vi "append_to_log.vi"(5 "data_type":T1, 7 "dims":T2, 8 "error in (no error)":errorcluster, 9 "Location":string, 10 "Data":variant, 11 "scan_hdf5_log in":refnum<class "scan_hdf5_log.lvclass">) -> (0 "error out":errorcluster, 3 "scan_hdf5_log out":refnum<class "scan_hdf5_log.lvclass">)   [LabVIEW 2015, in "scan_hdf5_log.lvclass"]
uses:
  scan_hdf5_log.lvclass
  Data Logger Class/data_dimensionality.ctl
  Data Logger Class/logger_data_types.ctl
  scan_hdf5_log.lvclass/scan_hdf5_log.ctl
  <vilib>/UPVI/lvhdf5/dataset.llb/Append Element(s) to Dataset (Variant).vi
  <vilib>/UPVI/lvhdf5/dataset.llb/Append Element(s) to Dataset.xnode
  <vilib>/UPVI/lvhdf5/library.llb/HDF5 Ref.ctl
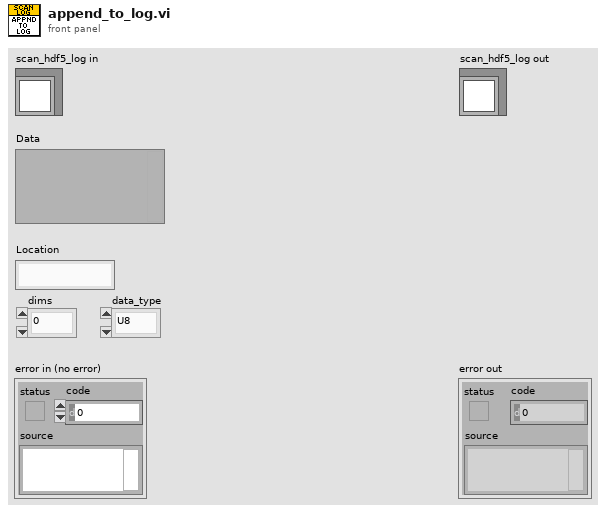
[diagram p1: front panel]
types:
  T1 = typedef "logger_data_types.ctl" = enum16{"U8", "I8", "U16", "I16", "U32", "I32", "DBL", "String"}
  T2 = typedef "data_dimensionality.ctl" = enum16{"0", "1", "2"}
  T3 = typedef "HDF5 Ref.ctl" = refnum<k1>
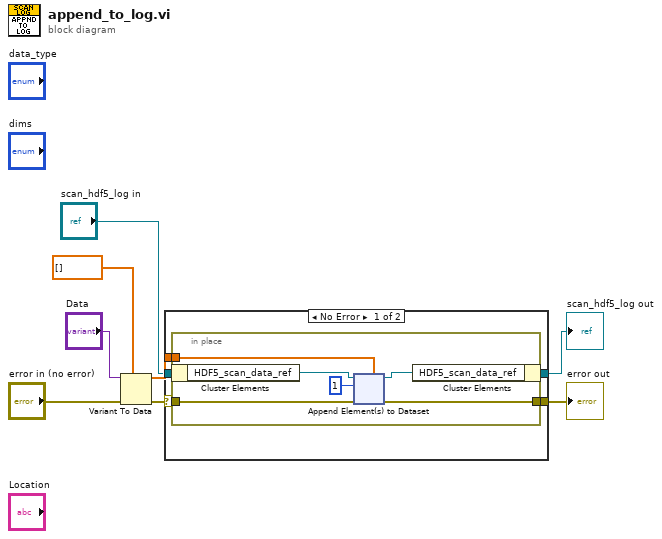
[diagram p0: block diagram]
diagram:
  n1 = Variant To Data(error in="error in (no error)", type=dbl[] [], Variant="Data") -> (data=w5:dbl[], error out=w4:errorcluster)
  n2 = case shown="No Error" w4 {
    selector: w4 -> [w11 w28]
    tunnel: w5 -> [w12 _]
    tunnel: "scan_hdf5_log in" -> [w13 w29]
    tunnel: [w10 w28] -> w2
    tunnel: [w9 w29] -> w1
    frame No Error {
      n3 = in-place {
        in-place-border: w12 -> [w16]
        in-place-border: w11 -> [w15]
        in-place-border: [w14] -> w10
        n4 = in-place-cluster #1(w13) -> ("HDF5_scan_data_ref"=w19:T3)
        n5 = xnode "Append Element(s) to Dataset"("Dimension to Extend (0)"=1, "HDF5 Dataset Ref"=w19, "error in (no error)"=w15, "Data Element(s)"=w16) -> ("HDF5 Dataset out"=w18:T3, "error out"=w14:errorcluster)  [unwired: 2 out]
        n6 = in-place-cluster #1("HDF5_scan_data_ref"=w18) -> (w9:refnum<class "scan_hdf5_log.lvclass">)
      }
    }
    frame Error {
    }
  }
  "error out" <- w2
  "scan_hdf5_log out" <- w1
